vi "SFC_WIPPVIRepair.vi"(5 ".NET:System.Data.DataSet":T1={"CaseSensitive"=FALSE, "Container"=refnum, "DataSetName"="", "DefaultViewManager"=refnum, "DesignMode"=FALSE, "EnforceConstraints"=FALSE, "ExtendedProperties"=refnum, "HasErrors"=FALSE, "IsInitialized"=FALSE, "Locale"=refnum, "Namespace"="", "Prefix"="", "Relations"=refnum, "RemotingFormat"=0, "SchemaSerializationMode"=1, "Site"=refnum, "Tables"=refnum} {"SchemaSerializationMode" items=["IncludeSchema"=1, "ExcludeSchema"=2]; "RemotingFormat" items=["Xml", "Binary"]}, 6 "UserNo":string, 7 "ProdLine":string, 8 "error in (no error)":errorcluster caption="错误输入（无错误）", 9 "RepCode":string, 10 "SID":string, 11 "Traceability 引用句柄":refnum<k24>) -> (0 "error out":errorcluster caption="错误输出", 2 "SFC_WIPPVIRepair":string, 3 "Traceability 引用句柄输出":refnum<k24>)   [LabVIEW 2014, in "Traceability.lvlib"]
uses:
  Traceability.lvlib
  Traceability.dll
  System.Data
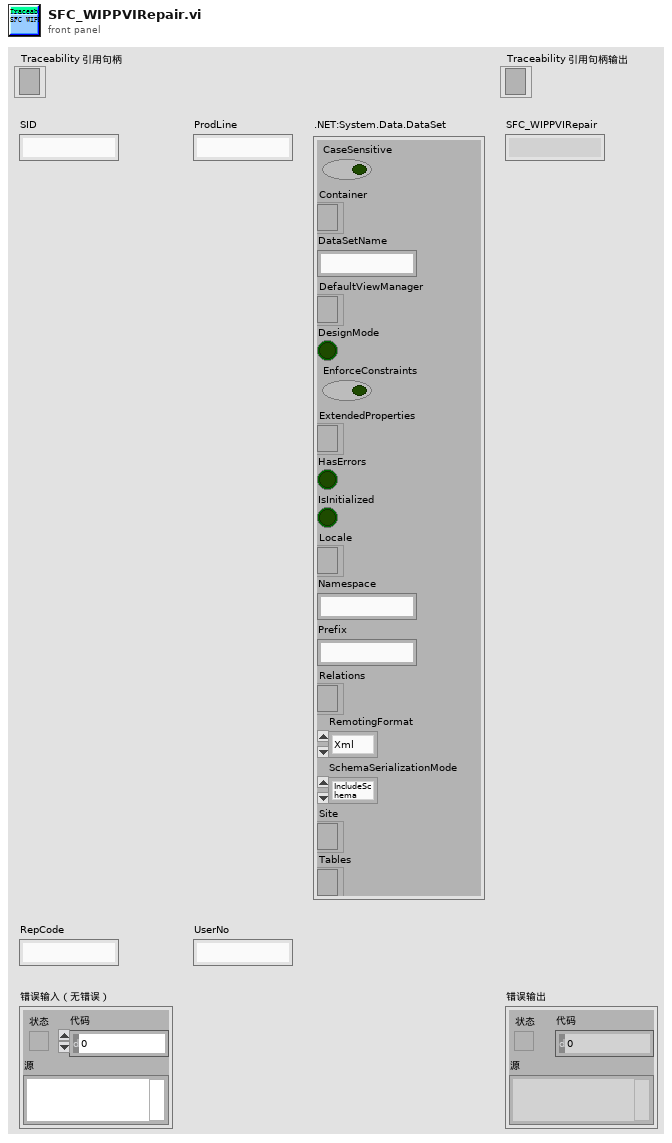
[diagram p1: front panel]
types:
  T1 = cluster{"CaseSensitive":bool, "Container":refnum<k24>, "DataSetName":string, "DefaultViewManager":refnum<k24>, "DesignMode":bool, "EnforceConstraints":bool, "ExtendedProperties":refnum<k24>, "HasErrors":bool, "IsInitialized":bool, "Locale":refnum<k24>, "Namespace":string, "Prefix":string, "Relations":refnum<k24>, "RemotingFormat":i32, "SchemaSerializationMode":i32, "Site":refnum<k24>, "Tables":refnum<k24>}
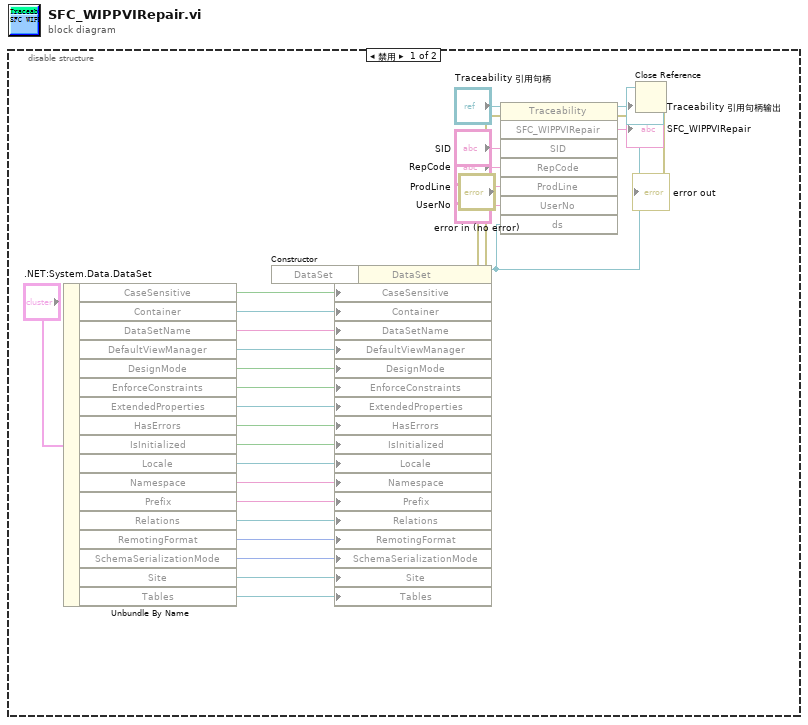
[diagram p0: block diagram]
diagram:
  n1 = disable-structure shown="禁用" {
    frame Disabled {
      n2 = Unbundle By Name(".NET:System.Data.DataSet") -> ("CaseSensitive"=w21:bool, "Container"=w20:refnum<k24>, "DataSetName"=w19:string, "DefaultViewManager"=w18:refnum<k24>, "DesignMode"=w17:bool, "EnforceConstraints"=w16:bool, "ExtendedProperties"=w15:refnum<k24>, "HasErrors"=w14:bool, "IsInitialized"=w13:bool, "Locale"=w12:refnum<k24>, "Namespace"=w11:string, "Prefix"=w10:string, "Relations"=w9:refnum<k24>, "RemotingFormat"=w8:i32, "SchemaSerializationMode"=w7:i32, "Site"=w6:refnum<k24>, "Tables"=w5:refnum<k24>)
      n3 = constructor class="DataSet"(error in="error in (no error)") -> (reference out=w25:refnum<k24>, error out=w24:errorcluster)  [unwired: 2 in, 1 out]
      n4 = property class="DataSet"(reference=w25, error in=w24, "CaseSensitive"=w21, "Container"=w20, "DataSetName"=w19, "DefaultViewManager"=w18, "DesignMode"=w17, "EnforceConstraints"=w16, "ExtendedProperties"=w15, "HasErrors"=w14, "IsInitialized"=w13, "Locale"=w12, "Namespace"=w11, "Prefix"=w10, "Relations"=w9, "RemotingFormat"=w8, "SchemaSerializationMode"=w7, "Site"=w6, "Tables"=w5) -> (reference out=w23:refnum<k24>, error out=w3:errorcluster)
      n5 = invoke class="Traceability" method="SFC_WIPPVIRepair"(reference="Traceability 引用句柄", error in=w3, "SID"="SID", "RepCode"="RepCode", "ProdLine"="ProdLine", "UserNo"="UserNo", "ds"=w23) -> (reference out=→"Traceability 引用句柄输出":refnum<k24>, error out=w2:errorcluster, "SFC_WIPPVIRepair"=→"SFC_WIPPVIRepair":string)  [unwired: 1 in, 5 out]
      n6 = Close Reference(reference=w23, error in (no error)=w2) -> (error out=→"error out":errorcluster)
    }
    frame Enabled {
    }
  }
